vi "visa_find_devices.vi"(8 "error in (no error)":errorcluster) -> (0 "error out":errorcluster, 2 "devices found string":string, 3 "find list":string[](array[string]))   [LabVIEW 2013, in "DDS.lvclass"]
uses:
  DDS.lvclass
panel:
  out "return count":u32
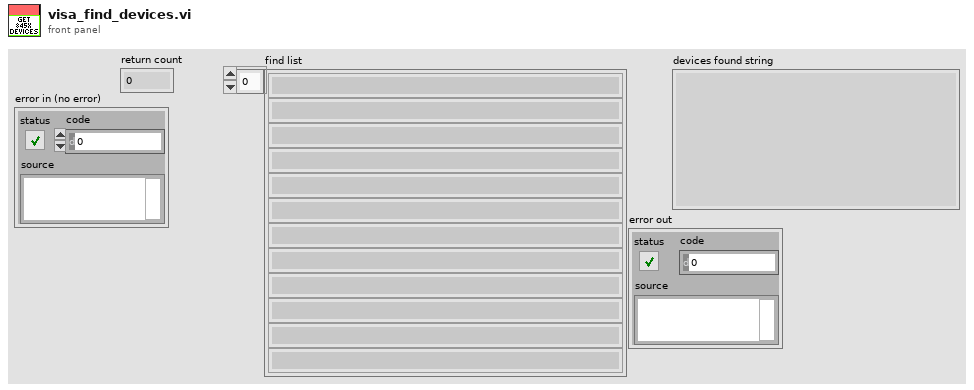
[diagram p1: front panel]
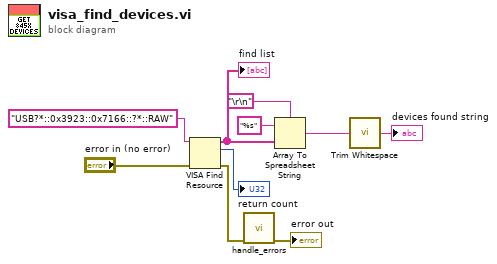
[diagram p0: block diagram]
diagram:
  n1 = VISA Find Resource(8:"error in (no error)", 11:"USB?*::0x3923::0x7166::?*::RAW" ("expression (\"?*\")")) -> (0:w2:errorcluster, 2:→"return count":u32, 3:w4:string[])  [unwired: 1 in]
  "find list" <- w4
  n2 = call "handle_errors.vi"("error in (no error)"=w2) -> ("error out"=→"error out":errorcluster)  [unwired: 14 in]
  n3 = Array To Spreadsheet String(delimiter (Tab)="\r\n", array=w4, 3:"%s" ("format string")) -> (spreadsheet string=w6:string)
  n4 = call <vilib>:"Trim Whitespace.vi"("string"=w6) -> ("trimmed string"=→"devices found string":string)  [unwired: 1 in]
